vi "Timer.vi"(8 "error in (no error)":errorcluster, 11 "cmd":T1) -> (0 "error out":errorcluster, 2 "string":string, 3 "Numeric":dbl format="%<%H:%M:%S>t")   [LabVIEW 2019]
uses:
  cmd_timer.ctl
  _ctrl/rw.ctl
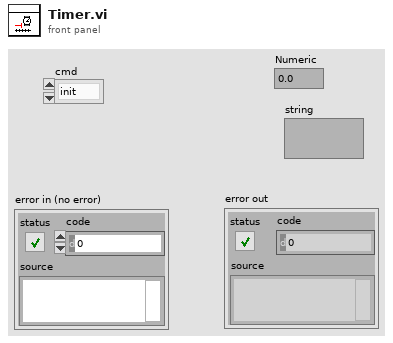
[diagram p1: front panel]
types:
  T1 = typedef "cmd_timer.ctl" = enum16{"init", "init_update", "run", "default", "update"}
  T2 = typedef "rw.ctl" = enum16{"read", "write"}
  T3 = typedef "ref_all.ctl" = cluster{"BP4610 Config":refnum<vi>, "DSP1950 Config":refnum<vi>, "2470-config":refnum<vi>, "cDAQ 9269 AO config":refnum<vi>, "cDAQ 9221 Config":refnum<vi>, "cDAQ-9467 Config":refnum<vi>, "Waveform":refnum<vi>, "DL950 wfm":refnum<vi>, "AI Graph":refnum<vi>, "AO_Wave-config":refnum<vi>, "DL950 items":refnum<vi>, "Volt":refnum<vi>, "Current":refnum<vi>, "AO_Level":refnum<vi>, "RC-Test Judgement ":refnum<vi>, "Log path":refnum<vi>, "시험명":refnum<vi>, "file renew[Hr]":refnum<vi>, "Breakdown-Spec":refnum<vi>, "paste":refnum<vi>, "copy":refnum<vi>, "DL950_config":refnum<vi>, "종료시간":refnum<vi>, "경과시간":refnum<vi>, "Apply":refnum<vi>, "DSP Config LV ":refnum<vi>, "Testconfig":refnum<vi>}
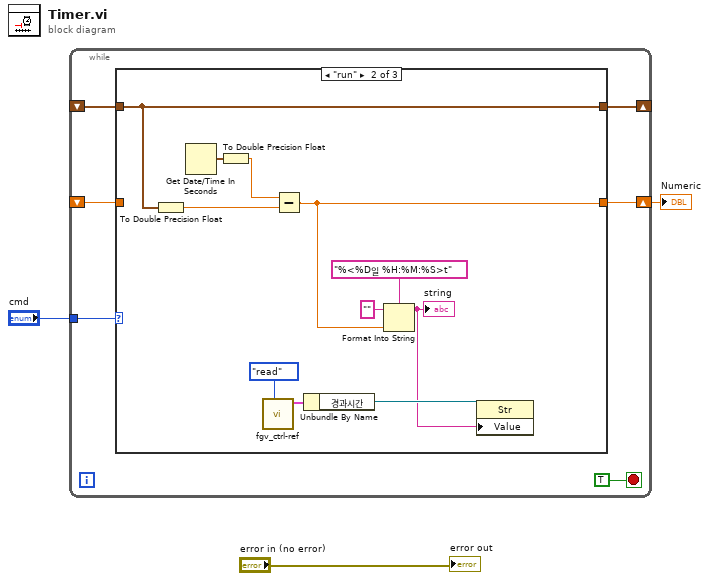
[diagram p0: block diagram]
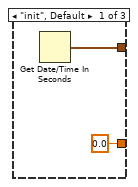
[diagram p2: hidden frame]
diagram:
  n1 = while {
    tunnel: "cmd" -> [w8]
    shift-right: [w7] -> _
    shift-left: _ -> [w6]
    shift-right: [w5] -> w1
    shift-left: _ -> [w4]
    stop <- TRUE stop-if-true
    n2 = case shown="\"run\"" w8 {
      tunnel: [w11 w20 w24] -> w7
      tunnel: w6 -> [_ w20 w24]
      tunnel: [0.0 w16 w23] -> w5
      tunnel: w4 -> [_ _ w23]
      frame "init", Default {
        n3 = Get Date/Time In Seconds() -> (seconds since 1Jan1904=w11:timestamp)
      }
      frame "run" {
        n4 = To Double Precision Float(number=w20) -> (double precision float=w19:dbl)
        n5 = Get Date/Time In Seconds() -> (seconds since 1Jan1904=w21:timestamp)
        n6 = To Double Precision Float(number=w21) -> (double precision float=w22:dbl)
        n7 = call "fgv_ctrl-ref.vi"("cmd"=rw."read") -> ("output cluster 2"=w14:T3)  [unwired: 9 in, 1 out]
        n8 = Subtract(x=w22, y=w19) -> (x-y=w16:dbl)
        n9 = Unbundle By Name(w14) -> ("경과시간"=w13:refnum<vi>)
        n10 = Format Into String(format string="%<%D일 %H:%M:%S>t", initial string="", w16) -> (resulting string=w12:string)  [unwired: 1 in, 1 out]
        "string" <- w12
        n11 = property class="Str"(reference=w13, "Value"=w12) -> ()  [unwired: 1 in, 2 out]
      }
      frame "default" {
      }
    }
  }
  "Numeric" <- w1
  "error out" <- "error in (no error)"
